vi "SecondPlatY.vi"(8 "错误输入（无错误）":errorcluster, 10 "CurrentY引用":refnum<vi>, 11 "Y引用":refnum<vi>) -> (0 "错误输出":errorcluster, 1 "Direction":i32, 2 "Step":i32, 3 "MotorNum":i32=6)   [LabVIEW 2011]
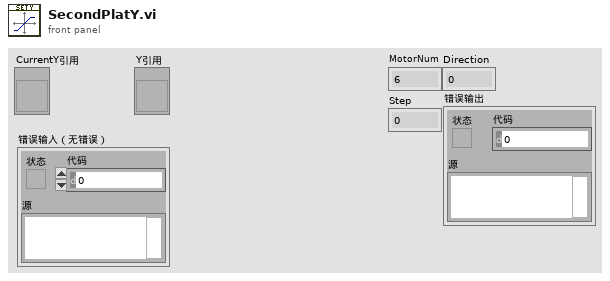
[diagram p1: front panel]
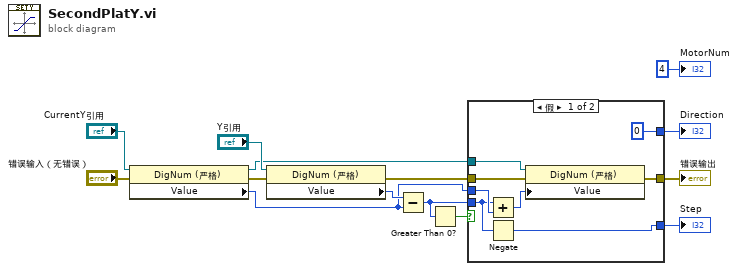
[diagram p0: block diagram]
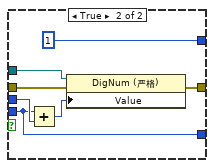
[diagram p2: hidden frame]
diagram:
  n1 = property on="属性节点" class="DigNum (严格)"(reference="CurrentY引用", error in="错误输入（无错误）") -> (reference out=w7:refnum<vi>, error out=w14:errorcluster, "Value"=w3:i32)
  n2 = property on="属性节点" class="DigNum (严格)"(reference="Y引用", error in=w14) -> (error out=w2:errorcluster, "Value"=w10:i32)  [unwired: 1 out]
  n3 = Subtract(x=w10, y=w3) -> (x-y=w8:i32)
  n4 = Greater Than 0?(x=w8) -> (x > 0?=w9:bool)
  n5 = case shown="假" w9 {
    tunnel: w8 -> [w18 w25]
    tunnel: [w22 w25] -> w5
    tunnel: w7 -> [w20 w28]
    tunnel: [0 1] -> w4
    tunnel: w3 -> [w19 w27]
    tunnel: [w16 w24] -> w1
    tunnel: w2 -> [w15 w23]
    frame False {
      n6 = Add(x=w18, y=w19) -> (x+y=w17:i32)
      n7 = Negate(x=w18) -> (-x=w22:i32)
      n8 = property on="属性节点" class="DigNum (严格)"(reference=w20, error in=w15, "Value"=w17) -> (error out=w16:errorcluster)  [unwired: 1 out]
    }
    frame True {
      n9 = Add(x=w25, y=w27) -> (x+y=w26:i32)
      n10 = property on="属性节点" class="DigNum (严格)"(reference=w28, error in=w23, "Value"=w26) -> (error out=w24:errorcluster)  [unwired: 1 out]
    }
  }
  "Step" <- w5
  "Direction" <- w4
  "错误输出" <- w1
  "MotorNum" <- 4
